vi "finishup.vi"(8 "error in (no error)":errorcluster, 11 "AnalysisResultsViewer in":refnum<class "AnalysisResultsViewer.lvclass">) -> (0 "error out":errorcluster, 3 "AnalysisResultsViewer out":refnum<class "AnalysisResultsViewer.lvclass">)   [LabVIEW 2011, in "Views.lvlib" / "Camera.lvlib" / "AnalysisResultsViewer.lvclass"]
uses:
  AnalysisResultsViewer.lvclass
  AnalysisResultsViewer.lvclass/AnalysisResultsViewer.ctl
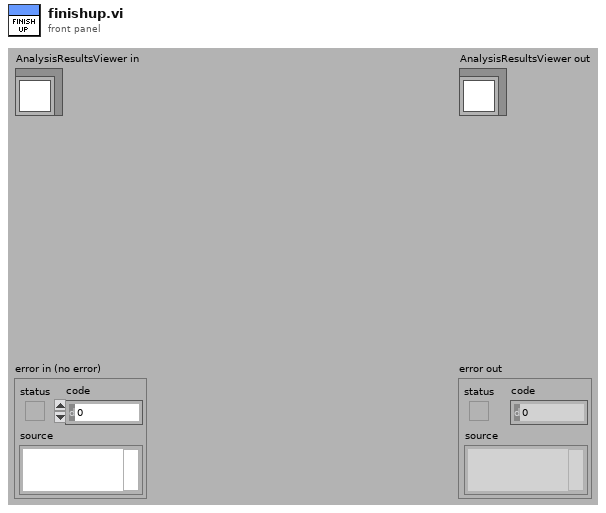
[diagram p1: front panel]
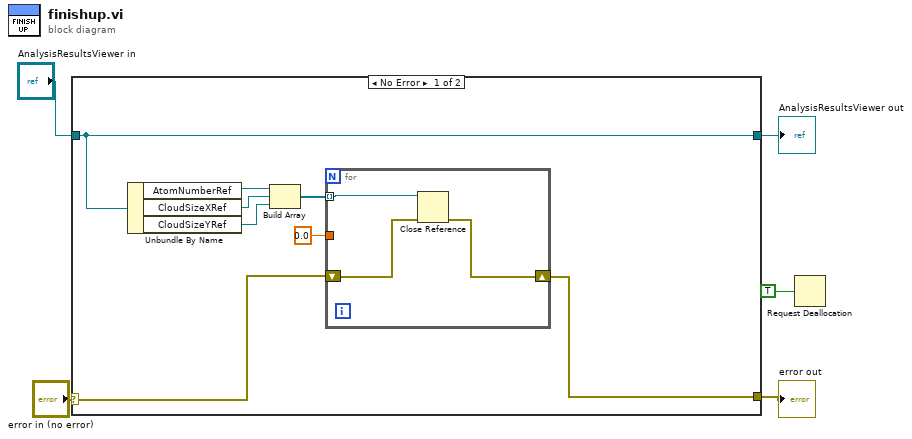
[diagram p0: block diagram]
diagram:
  n1 = case shown="No Error" "error in (no error)" {
    selector: "error in (no error)" -> [w8 w18]
    tunnel: [w7 w18] -> w4
    tunnel: [w6 w17] -> w2
    tunnel: "AnalysisResultsViewer in" -> [w6 w17]
    frame No Error {
      n2 = Unbundle By Name(w6) -> ("AtomNumberRef"=w13:refnum<vi>, "CloudSizeXRef"=w12:refnum<vi>, "CloudSizeYRef"=w11:refnum<vi>)
      n3 = Build Array(w13, w12, w11) -> (w10:refnum<vi>[])
      n4 = for {
        tunnel: w10 -> [w16] mode=indexing
        tunnel: 0.0 -> [_]
        shift-right: [w14] -> w7
        shift-left: w8 -> [w15]
        n5 = Close Reference(reference=w16, error in (no error)=w15) -> (error out=w14:errorcluster)
      }
    }
    frame Error {
    }
  }
  "error out" <- w4
  "AnalysisResultsViewer out" <- w2
  n6 = Request Deallocation(TRUE ("flag")) -> ()
